vi "Insert.vi"(6 "commandTimeout":i32, 7 "SqlMapper in":refnum<class "SqlMapper.lvclass">, 8 "error in (no error)":errorcluster, 9 "DynamicParameters":refnum<class "DynamicParameters.lvclass">, 10 "tableName":string, 11 "SQLConnection in":refnum<class "SQLConnection.lvclass">) -> (0 "error out":errorcluster, 2 "id":variant, 3 "SQLConnection out":refnum<class "SQLConnection.lvclass">, 5 "SqlMapper out":refnum<class "SqlMapper.lvclass">)   [LabVIEW 2018]
uses:
  SQLConnection.lvclass
  Dapper/SqlMapper/SqlMapper.lvclass
  Dapper/DynamicParameters/DynamicParameters.lvclass
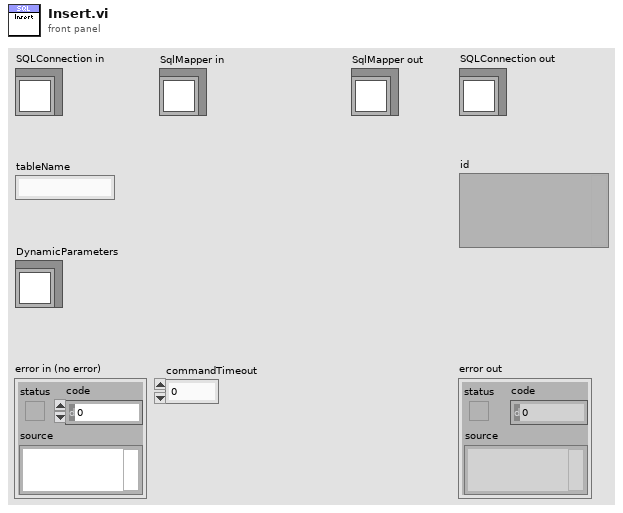
[diagram p1: front panel]
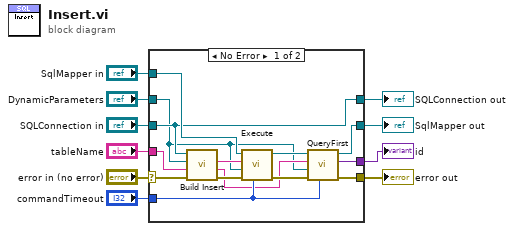
[diagram p0: block diagram]
diagram:
  n1 = case shown="No Error" "error in (no error)" {
    selector: "error in (no error)" -> [w22 w27]
    tunnel: [w18 w27] -> w2
    tunnel: [w12 w26] -> w5
    tunnel: "SQLConnection in" -> [w12 w26]
    tunnel: "SqlMapper in" -> [w24 w25]
    tunnel: "DynamicParameters" -> [w11 _]
    tunnel: [w14 _] -> w3
    tunnel: "commandTimeout" -> [w17 _]
    tunnel: [w15 w25] -> w4
    tunnel: "tableName" -> [w20 _]
    frame No Error {
      n2 = call-dynamic "Build Insert.vi"("error in (no error)"=w22, "tableName"=w20, "DynamicParameters in"=w11, "SQLConnection in"=w12) -> ("error out"=w23:errorcluster, "LastIdentityQuery"=w13:string, "InsertStatement"=w21:string)  [unwired: 5 in]
      n3 = call-dynamic "Execute.vi"("commandTimeout"=w17, "error in (no error)"=w23, "DynamicParameters"=w11, "sql"=w21, "SqlMapper in"=w24) -> ("error out"=w19:errorcluster, "SqlMapper out"=w16:refnum<class "SqlMapper.lvclass">)  [unwired: 4 in, 1 out]
      n4 = call-dynamic "QueryFirst.vi"("commandTimeout in"=w17, "error in (no error)"=w19, "DynamicParameters in"=w11, "sql"=w13, "SqlMapper in"=w16) -> ("error out"=w18:errorcluster, "Value"=w14:variant, "SqlMapper out"=w15:refnum<class "SqlMapper.lvclass">)  [unwired: 4 in]
    }
    frame Error {
    }
  }
  "error out" <- w2
  "SQLConnection out" <- w5
  "id" <- w3
  "SqlMapper out" <- w4
